vi "1.vi"() -> ()   [LabVIEW 2020]
panel:
  in  "stop":bool
  out "Waveform Chart":dbl(graph)
  in  "dx":dbl
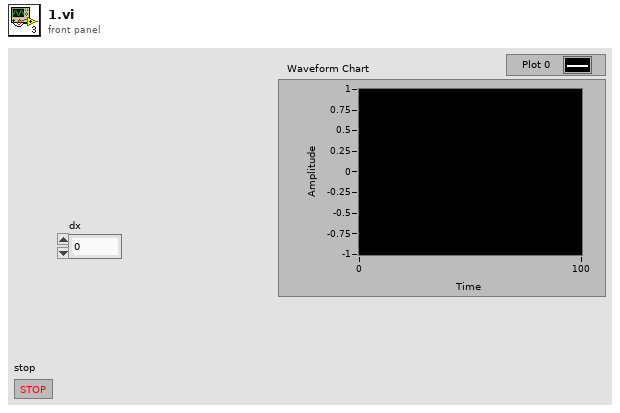
[diagram p1: front panel]
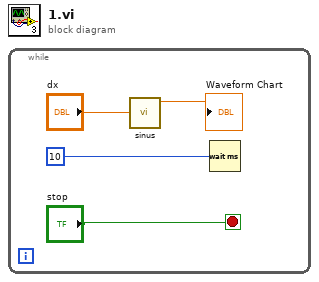
[diagram p0: block diagram]
diagram:
  n1 = while {
    stop <- "stop" stop-if-true
    n2 = call "sinus.vi"("dx"="dx") -> ("sin(x)"=→"Waveform Chart":dbl)  [unwired: 9 in, 1 out]
    n3 = Wait (ms)(milliseconds to wait=u32 10 ("millisecond timer value")) -> ()  [unwired: 1 out]
  }
